vi "Pressure Trigger Find v0.vi"(6 "Iteration":i32, 7 "Threshold":dbl, 10 "Current Value":dbl, 11 "ROI":dbl format="%#_24g") -> (1 "Triggered?":bool, 3 "Peak Value":dbl)   [LabVIEW 2017]
doc: "Rememer to initialize with a 0 three times!"
panel:
  out "Last Value":dbl
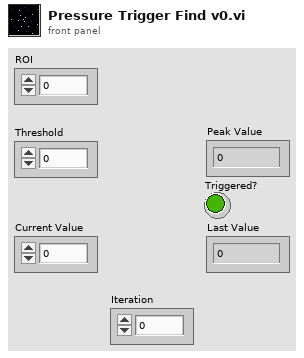
[diagram p1: front panel]
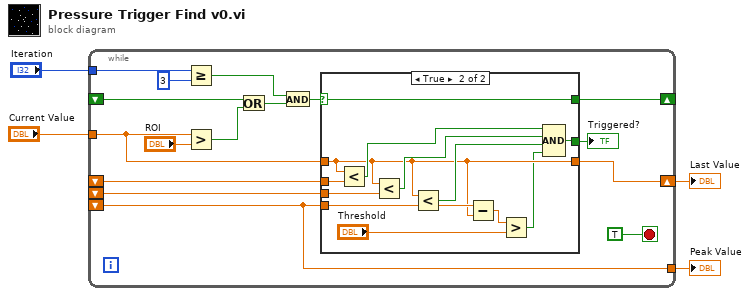
[diagram p0: block diagram]
diagram:
  n1 = while {
    shift-right: [w18] -> w4
    shift-left: _ -> [w20]
    shift-left: _ -> [w5]
    shift-left: _ -> [w19]
    shift-right: [w17] -> _
    shift-left: _ -> [w15]
    tunnel: "Current Value" -> [w14]
    tunnel: "Iteration" -> [w10]
    tunnel: [w5] -> w1
    stop <- TRUE stop-if-true
    n2 = Greater Or Equal?(x=w10, y=3) -> (x >= y?=w6:bool)
    n3 = Greater?(x=w14, y="ROI") -> (0:w16:bool)
    n4 = Or(x=w15, y=w16) -> (x .or. y?=w8:bool)
    n5 = And(x=w6, y=w8) -> (x .and. y?=w7:bool)
    n6 = case shown="True" w7 {
      selector: w7 -> [w21 w26]
      tunnel: w14 -> [w22 w24]
      tunnel: w20 -> [_ w34]
      tunnel: w19 -> [_ w33]
      tunnel: w5 -> [_ w25]
      tunnel: [w22 w24] -> w18
      tunnel: [_ w30] -> w13
      tunnel: [w21 w26] -> w17
      frame False {
      }
      frame True {
        n7 = Less?(x=w24, y=w34) -> (x < y?=w29:bool)
        n8 = Less?(x=w24, y=w33) -> (x < y?=w28:bool)
        n9 = Less?(x=w24, y=w25) -> (x < y?=w27:bool)
        n10 = Subtract(x=w25, y=w24) -> (x-y=w32:dbl)
        n11 = Greater?(x=w32, y="Threshold") -> (0:w23:bool)
        n12 = Compound Arithmetic op=AND(w29, w28, w27, w23) -> (w30:bool)
      }
    }
    "Triggered?" <- w13
  }
  "Last Value" <- w4
  "Peak Value" <- w1
